vi "Get Translated Item Text.vi"(8 "error in (no error)":errorcluster, 9 "LangIndex (0)":i32, 10 "ItemName":string, 11 "GObject in":refnum<class "GObject.lvclass">) -> (0 "error out":errorcluster, 1 "Found?":bool, 2 "Translated Text (ASCII)":string, 3 "GObject out":refnum<class "GObject.lvclass">)   [LabVIEW 2013, in "SET Project Data.lvlib" / "GObject.lvclass"]
uses:
  GObject.lvclass
  GObject.lvclass/GObject.ctl
  Resource Data Class/Resource Data.lvclass
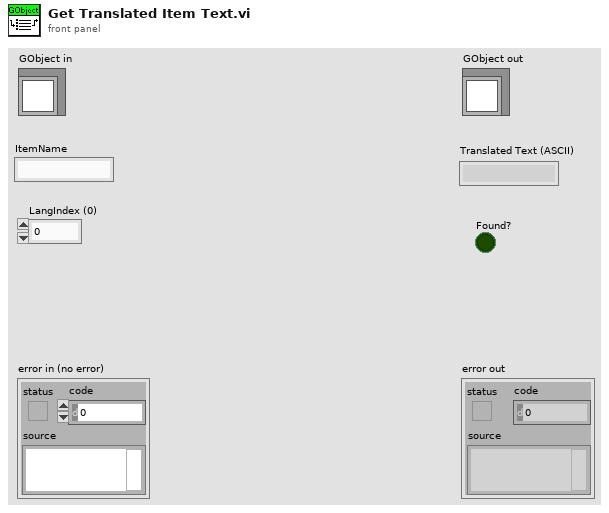
[diagram p1: front panel]
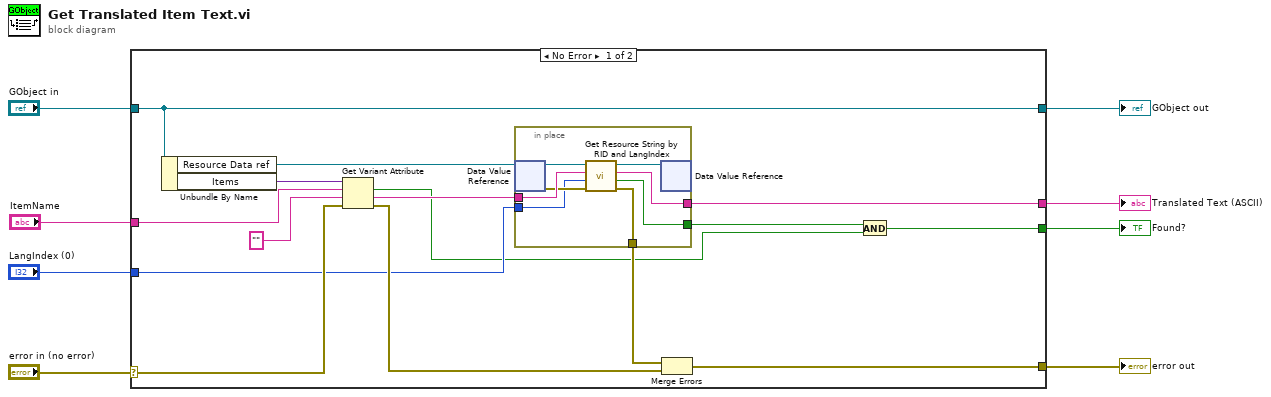
[diagram p0: block diagram]
diagram:
  n1 = case shown="No Error" "error in (no error)" {
    selector: "error in (no error)" -> [w20 w33]
    tunnel: [w14 w33] -> w7
    tunnel: [w23 w32] -> w5
    tunnel: "GObject in" -> [w23 w32]
    tunnel: "ItemName" -> [w21 _]
    tunnel: "LangIndex (0)" -> [w13 _]
    tunnel: [w12 _] -> w2
    tunnel: [w9 _] -> w1
    frame No Error {
      n2 = Unbundle By Name(w23) -> ("Resource Data ref"=w19:refnum<data-value>, "Items"=w22:variant)
      n3 = Get Variant Attribute(Variant=w22, name=w21, default value (empty Variant)="", error in=w20) -> (found=w10:bool, value=w17:string, error out=w16:errorcluster)  [unwired: 1 out]
      n4 = in-place {
        in-place-border: w17 -> [w29]
        in-place-border: [w27] -> w11
        in-place-border: [w26] -> w15
        in-place-border: w13 -> [w25]
        in-place-border: [w24] -> w12
        n5 = in-place-dvr #1(w19) -> (w31:refnum<class "Resource Data.lvclass">, w28:errorcluster)
        n6 = call "Get Resource String by RID and LangIndex.vi"("error in (no error)"=w28, "LangIndex (0)"=w25, "RID"=w29, "LangFile in"=w31) -> ("error out"=w26:errorcluster, "Found?"=w27:bool, "Translated Text (ASCII)"=w24:string, "LangFile out"=w30:refnum<class "Resource Data.lvclass">)  [unwired: 4 in]
        n7 = in-place-dvr #1(w30) -> ()  [unwired: 2 out]
      }
      n8 = Merge Errors(w15, w16) -> (w14:errorcluster)
      n9 = And(x=w11, y=w10) -> (x .and. y?=w9:bool)
    }
    frame Error {
    }
  }
  "error out" <- w7
  "GObject out" <- w5
  "Translated Text (ASCII)" <- w2
  "Found?" <- w1
